vi "sanitize string.vi"(4 "string in":string) -> (1 "validated string":string)   [LabVIEW 2025, in "Error Wrapper.lvlib"]
uses:
  Error Wrapper.lvlib
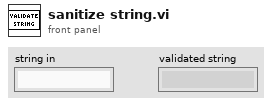
[diagram p1: front panel]
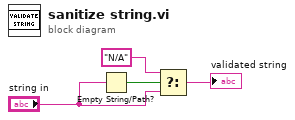
[diagram p0: block diagram]
diagram:
  n1 = Empty String/Path?(string/path="string in") -> (empty?=w1:bool)
  n2 = Select(t="N/A", s=w1, f="string in") -> (s? t:f=→"validated string":string)
